vi "xGlobal Data.vi"() -> ()   [LabVIEW 2016, in "SuperActor.lvlib" / "SuperActor.lvclass"]
uses:
  SuperActor.lvclass
panel:
  in  "Cfg Path":path=path "c:/exscalabar/cfg/exscalabar.ini"
  in  "Log Path":path=path "u:/exscalabar/logs"
  in  "Cfg":string="Cfg Session"
  in  "Log":string="Log Session"
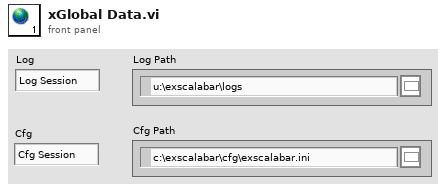
[diagram p1: front panel]
diagram:
